vi "main.vi"() -> ()   [LabVIEW 2023]
uses:
  #typedef_state.ctl
  #typedef_caffeetype.ctl
  #typedef_data.ctl
  #typedef_action.ctl
  <vilib>/Utility/file.llb/Write Delimited Spreadsheet (string).vi
panel:
  in  "Caffee Mocha":bool
  in  "Caffee Latte":bool
  in  "Espresso Macchiato":bool
  in  "Espresso":bool
  in  "stop":bool
  out "Whipped Cream":bool
  out "Chocolate Syrup":bool
  out "Milk Foam":bool
  out "Steamed Milk":bool
  out "Espresso":bool
  # "Wybierz kawe:"
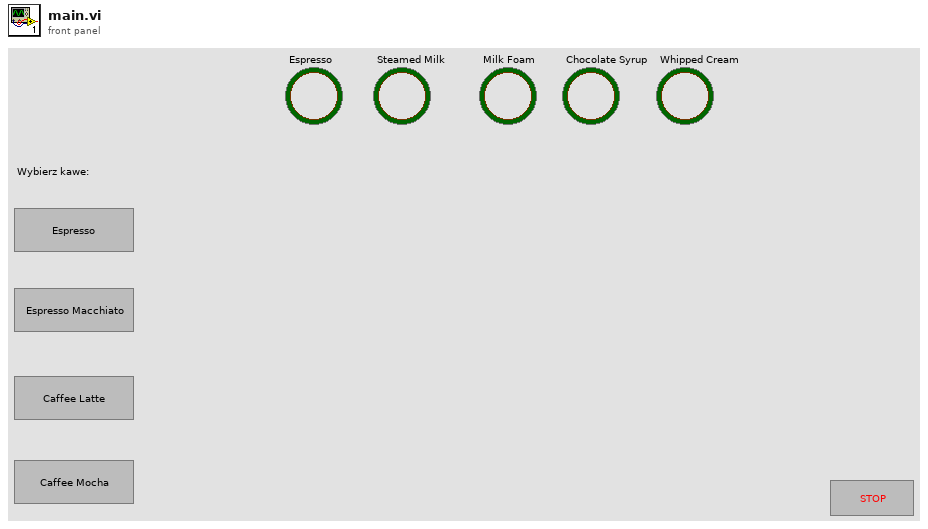
[diagram p1: front panel]
types:
  T1 = typedef "#typedef_caffeetype.ctl" = enum16{"Espresso", "Espresso Macchiato", "Caffee Latte", "Caffee Mocha"}
  T2 = typedef "#typedef_state.ctl" = enum16{"Inicializing", "Idle", "Whipped Cream", "Chocolate Syrup", "Milk Foam", "Steamed Milk", "Espresso", "Stop"}
  T3 = typedef "#typedef_data.ctl" = cluster{"Caffee Type":enum16{"Espresso", "Espresso Macchiato", "Caffee Latte", "Caffee Mocha"}, "Espresso":bool, "Steamed Milk":bool, "Milk Foam":bool, "Chocolate Syrup":bool, "Whipped Cream":bool, "Time reset?":bool}
  T4 = enum16{"Espresso", "Espresso Macchiato", "Caffee Latte", "Caffee Mocha"}
  T5 = typedef "#typedef_action.ctl" = enum16{"Pause", "Reset", "Run"}
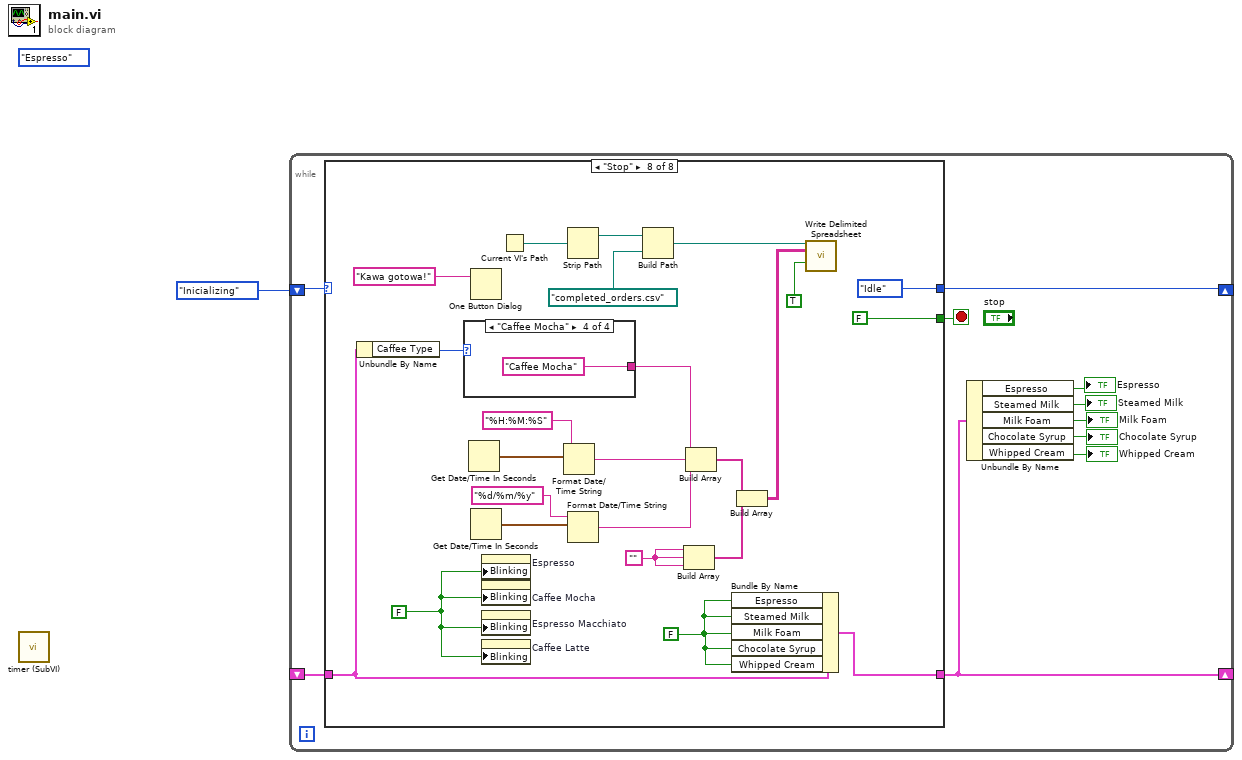
[diagram p0: block diagram]
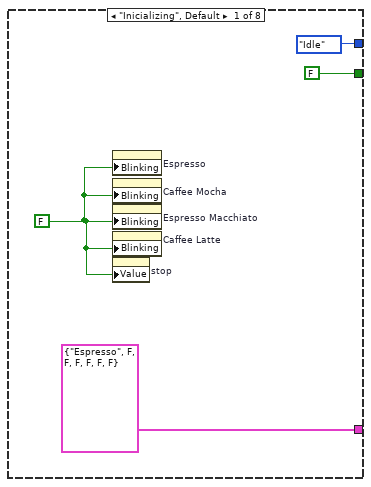
[diagram p2: hidden frame]
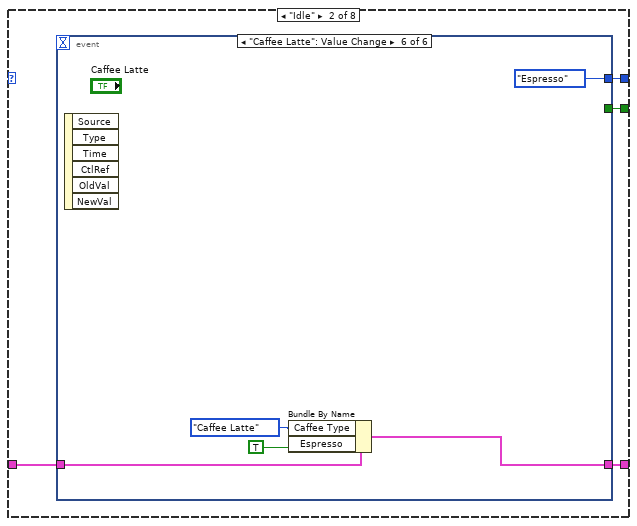
[diagram p3: hidden frame]
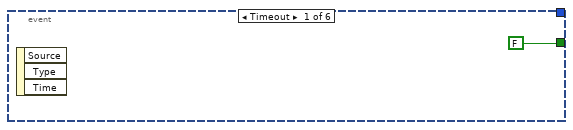
[diagram p4: hidden frame]
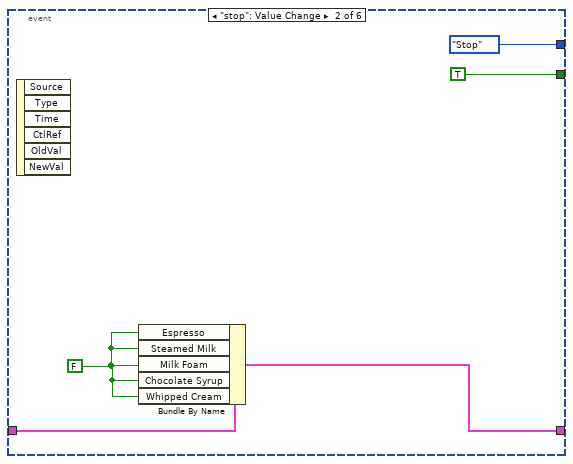
[diagram p5: hidden frame]
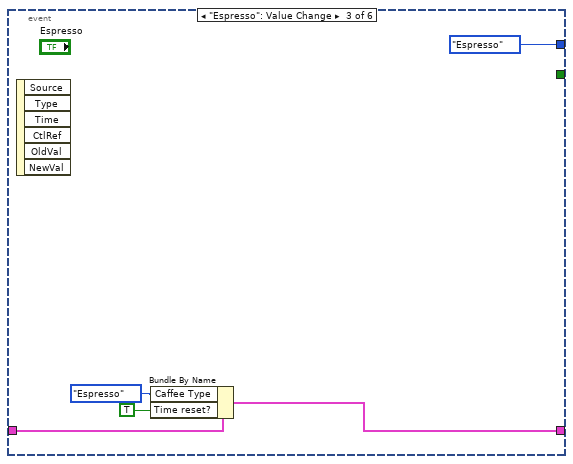
[diagram p6: hidden frame]
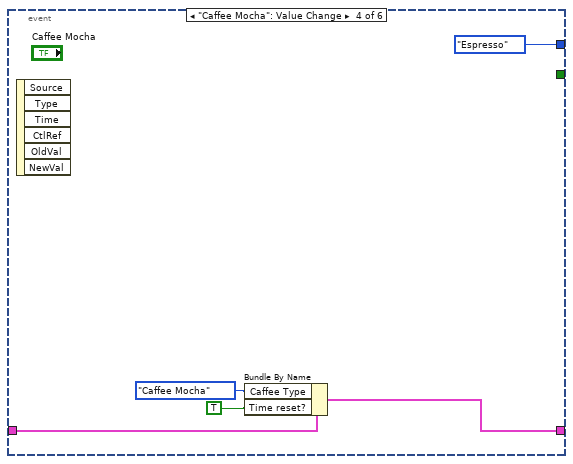
[diagram p7: hidden frame]
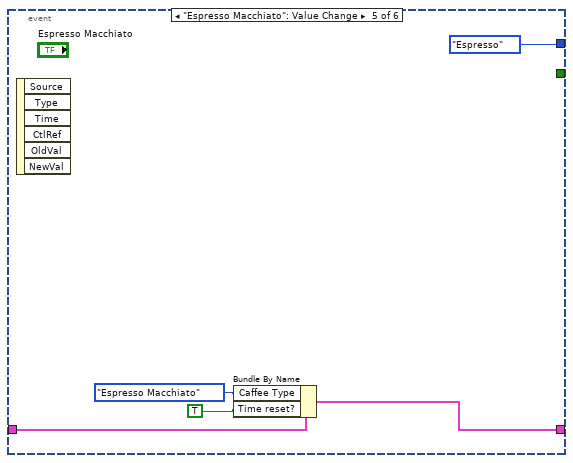
[diagram p8: hidden frame]
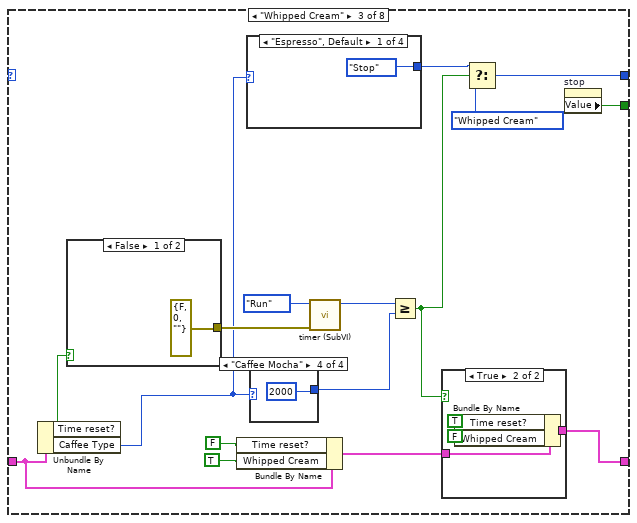
[diagram p9: hidden frame]
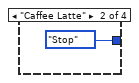
[diagram p11: hidden frame]
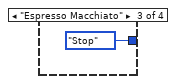
[diagram p12: hidden frame]
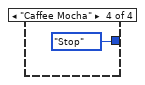
[diagram p13: hidden frame]
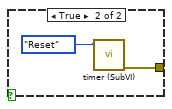
[diagram p14: hidden frame]
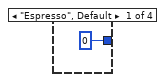
[diagram p15: hidden frame]
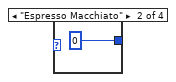
[diagram p16: hidden frame]
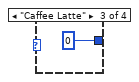
[diagram p17: hidden frame]
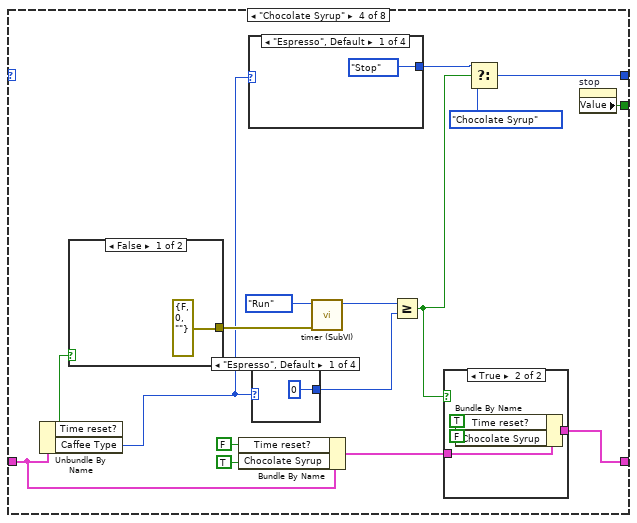
[diagram p18: hidden frame]
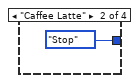
[diagram p20: hidden frame]
diagram:
  (unwired) #typedef_caffeetype."Espresso" ("Caffee Type")
  n1 = call "timer (SubVI).vi"() -> ()  [unwired: 10 in, 2 out]
  n2 = while {
    shift-right: [w10] -> _
    shift-left: #typedef_state."Inicializing" ("State") -> [w11]
    shift-right: [w7] -> _
    shift-left: _ -> [w8]
    stop <- w9 stop-if-true
    n3 = case shown="\"Stop\"" w11 {
      tunnel: [T3 {"Caffee Type"=enum."Espresso", "Espresso"=FALSE, "Steamed Milk"=FALSE, "Milk Foam"=FALSE, "Chocolate Syrup"=FALSE, "Whipped Cream"=FALSE, "Time reset?"=FALSE} ("Data") w16 w49 w80 w114 w144 w177 w230] -> w7
      tunnel: [#typedef_state."Idle" ("State") w18 w51 w82 w115 w146 w183 #typedef_state."Idle" ("State")] -> w10
      tunnel: [FALSE w19 w48 w79 w112 w143 w176 FALSE] -> w9
      tunnel: w8 -> [_ w17 w50 w81 w113 w145 w189 w220]
      frame "Inicializing", Default {
        w12 = FALSE ("stop")
        n4 = property on="Espresso" class="Bool"("Blinking"=w12) -> ()  [unwired: 2 in, 2 out]
        n5 = property on="Caffee Mocha" class="Bool"("Blinking"=w12) -> ()  [unwired: 2 in, 2 out]
        n6 = property on="Espresso Macchiato" class="Bool"("Blinking"=w12) -> ()  [unwired: 2 in, 2 out]
        n7 = property on="Caffee Latte" class="Bool"("Blinking"=w12) -> ()  [unwired: 2 in, 2 out]
        n8 = property on="stop" class="Bool (strict)"("Value"=w12) -> ()  [unwired: 2 in, 2 out]
      }
      frame "Idle" {
        n9 = event shown="[5] \"Caffee Latte\": Value Change" {
          selector: _ -> [_ _ _ _ _ _]
          dyn-events: _ -> [_ _ _ _ _ _]
          timeout: _ -> [_ _ _ _ _ _]
          tunnel: [FALSE TRUE _ _ _ _] -> w19
          tunnel: [_ #typedef_state."Stop" ("State") #typedef_state."Espresso" ("State") #typedef_state."Espresso" ("State") #typedef_state."Espresso" ("State") #typedef_state."Espresso" ("State")] -> w18
          tunnel: w17 -> [_ w23 w29 w33 w39 w44]
          tunnel: [_ w21 w27 w32 w38 w43] -> w16
          event Timeout {
            n10 = event-data() -> ()  [unwired: 1 in, 3 out]
          }
          event "stop": Value Change {
            w22 = FALSE ("Espresso")
            n11 = event-data() -> ()  [unwired: 1 in, 6 out]
            n12 = Bundle By Name(cluster=w23, "Espresso"=w22, "Steamed Milk"=w22, "Milk Foam"=w22, "Chocolate Syrup"=w22, "Whipped Cream"=w22) -> (w21:T3)
          }
          event "Espresso": Value Change {
            n13 = event-data() -> ()  [unwired: 1 in, 6 out]
            n14 = Bundle By Name(cluster=w29, "Caffee Type"=T4."Espresso", "Time reset?"=TRUE) -> (w27:T3)
          }
          event "Caffee Mocha": Value Change {
            n15 = event-data() -> ()  [unwired: 1 in, 6 out]
            n16 = Bundle By Name(cluster=w33, "Caffee Type"=T4."Caffee Mocha", "Time reset?"=TRUE) -> (w32:T3)
          }
          event "Espresso Macchiato": Value Change {
            n17 = event-data() -> ()  [unwired: 1 in, 6 out]
            n18 = Bundle By Name(cluster=w39, "Caffee Type"=T4."Espresso Macchiato", "Time reset?"=TRUE) -> (w38:T3)
          }
          event "Caffee Latte": Value Change {
            n19 = event-data() -> ()  [unwired: 1 in, 6 out]
            n20 = Bundle By Name(cluster=w44, "Caffee Type"=T4."Caffee Latte", "Espresso"=TRUE) -> (w43:T3)
          }
        }
      }
      frame "Whipped Cream" {
        n21 = Unbundle By Name(w50) -> ("Time reset?"=w59:bool, "Caffee Type"=w56:T4)
        n22 = case shown="False" w59 {
          tunnel: [errorcluster {"status"=FALSE, "code"=0, "source"=""} ("error out") w73] -> w61
          frame False {
          }
          frame True {
            n23 = call "timer (SubVI).vi"("Action"=#typedef_action."Reset") -> ("error out"=w73:errorcluster)  [unwired: 9 in, 1 out]
          }
        }
        n24 = Bundle By Name(cluster=w50, "Time reset?"=FALSE, "Whipped Cream"=TRUE) -> (w52:T3)
        n25 = case shown="\"Espresso\", Default" w56 {
          tunnel: [#typedef_state."Stop" ("State") #typedef_state."Stop" ("State") #typedef_state."Stop" ("State") #typedef_state."Stop" ("State")] -> w55
          frame "Espresso", Default {
          }
          frame "Caffee Latte" {
          }
          frame "Espresso Macchiato" {
          }
          frame "Caffee Mocha" {
          }
        }
        n26 = case shown="\"Caffee Mocha\"" w56 {
          tunnel: [0 0 0 2000] -> w58
          frame "Espresso", Default {
          }
          frame "Espresso Macchiato" {
          }
          frame "Caffee Latte" {
          }
          frame "Caffee Mocha" {
          }
        }
        n27 = call "timer (SubVI).vi"("error in (no error)"=w61, "Action"=#typedef_action."Run") -> ("Numeric"=w60:u32)  [unwired: 8 in, 1 out]
        n28 = Greater Or Equal?(x=w60, y=w58) -> (x >= y?=w53:bool)
        n29 = case shown="True" w53 {
          tunnel: w52 -> [w62 w66]
          tunnel: [w62 w63] -> w49
          frame False {
          }
          frame True {
            n30 = Bundle By Name(cluster=w66, "Time reset?"=TRUE, "Whipped Cream"=FALSE ("Espresso")) -> (w63:T3)
          }
        }
        n31 = Select(t=w55, s=w53, f=#typedef_state."Whipped Cream" ("State")) -> (s? t:f=w51:T2)
        n32 = property on="stop" class="Bool (strict)"() -> ("Value"=w48:bool)  [unwired: 2 in, 2 out]
      }
      frame "Chocolate Syrup" {
        n33 = Unbundle By Name(w81) -> ("Time reset?"=w91:bool, "Caffee Type"=w87:T4)
        n34 = case shown="False" w91 {
          tunnel: [errorcluster {"status"=FALSE, "code"=0, "source"=""} ("error out") w105] -> w93
          frame False {
          }
          frame True {
            n35 = call "timer (SubVI).vi"("Action"=#typedef_action."Reset") -> ("error out"=w105:errorcluster)  [unwired: 9 in, 1 out]
          }
        }
        n36 = Bundle By Name(cluster=w81, "Time reset?"=FALSE, "Chocolate Syrup"=TRUE) -> (w83:T3)
        n37 = case shown="\"Espresso\", Default" w87 {
          tunnel: [#typedef_state."Stop" ("State") #typedef_state."Stop" ("State") #typedef_state."Stop" ("State") #typedef_state."Steamed Milk" ("State")] -> w86
          frame "Espresso", Default {
          }
          frame "Caffee Latte" {
          }
          frame "Espresso Macchiato" {
          }
          frame "Caffee Mocha" {
          }
        }
        n38 = case shown="\"Espresso\", Default" w87 {
          tunnel: [0 0 0 2000] -> w89
          frame "Espresso", Default {
          }
          frame "Espresso Macchiato" {
          }
          frame "Caffee Latte" {
          }
          frame "Caffee Mocha" {
          }
        }
        n39 = call "timer (SubVI).vi"("error in (no error)"=w93, "Action"=#typedef_action."Run") -> ("Numeric"=w92:u32)  [unwired: 8 in, 1 out]
        n40 = Greater Or Equal?(x=w92, y=w89) -> (x >= y?=w84:bool)
        n41 = case shown="True" w84 {
          tunnel: w83 -> [w94 w98]
          tunnel: [w94 w95] -> w80
          frame False {
          }
          frame True {
            n42 = Bundle By Name(cluster=w98, "Time reset?"=TRUE, "Chocolate Syrup"=FALSE ("Espresso")) -> (w95:T3)
          }
        }
        n43 = Select(t=w86, s=w84, f=#typedef_state."Chocolate Syrup" ("State")) -> (s? t:f=w82:T2)
        n44 = property on="stop" class="Bool (strict)"() -> ("Value"=w79:bool)  [unwired: 2 in, 2 out]
      }
      frame "Milk Foam" {
        n45 = Unbundle By Name(w113) -> ("Time reset?"=w123:bool, "Caffee Type"=w120:T4)
        n46 = case shown="True" w123 {
          tunnel: [errorcluster {"status"=FALSE, "code"=0, "source"=""} ("error out") w137] -> w125
          frame False {
          }
          frame True {
            n47 = call "timer (SubVI).vi"("Action"=#typedef_action."Reset") -> ("error out"=w137:errorcluster)  [unwired: 9 in, 1 out]
          }
        }
        n48 = case shown="\"Espresso Macchiato\"" w120 {
          tunnel: [#typedef_state."Stop" ("State") #typedef_state."Stop" ("State") #typedef_state."Stop" ("State") #typedef_state."Stop" ("State")] -> w119
          frame "Espresso", Default {
          }
          frame "Caffee Latte" {
          }
          frame "Espresso Macchiato" {
          }
          frame "Caffee Mocha" {
          }
        }
        n49 = case shown="\"Caffee Latte\"" w120 {
          tunnel: [0 2000 2000 0] -> w122
          frame "Espresso", Default {
          }
          frame "Espresso Macchiato" {
          }
          frame "Caffee Latte" {
          }
          frame "Caffee Mocha" {
          }
        }
        n50 = Bundle By Name(cluster=w113, "Time reset?"=FALSE, "Milk Foam"=TRUE) -> (w116:T3)
        n51 = call "timer (SubVI).vi"("error in (no error)"=w125, "Action"=#typedef_action."Run") -> ("Numeric"=w124:u32)  [unwired: 8 in, 1 out]
        n52 = Greater Or Equal?(x=w124, y=w122) -> (x >= y?=w117:bool)
        n53 = case shown="True" w117 {
          tunnel: w116 -> [w126 w130]
          tunnel: [w126 w127] -> w114
          frame False {
          }
          frame True {
            n54 = Bundle By Name(cluster=w130, "Time reset?"=TRUE, "Milk Foam"=FALSE ("Espresso")) -> (w127:T3)
          }
        }
        n55 = Select(t=w119, s=w117, f=#typedef_state."Milk Foam" ("State")) -> (s? t:f=w115:T2)
        n56 = property on="stop" class="Bool (strict)"() -> ("Value"=w112:bool)  [unwired: 2 in, 2 out]
      }
      frame "Steamed Milk" {
        n57 = Unbundle By Name(w145) -> ("Time reset?"=w155:bool, "Caffee Type"=w151:T4)
        n58 = case shown="True" w155 {
          tunnel: [errorcluster {"status"=FALSE, "code"=0, "source"=""} ("error out") w169] -> w157
          frame False {
          }
          frame True {
            n59 = call "timer (SubVI).vi"("Action"=#typedef_action."Reset") -> ("error out"=w169:errorcluster)  [unwired: 9 in, 1 out]
          }
        }
        n60 = Bundle By Name(cluster=w145, "Time reset?"=FALSE, "Steamed Milk"=TRUE) -> (w147:T3)
        n61 = case shown="\"Caffee Latte\"" w151 {
          tunnel: [0 0 8000 2000] -> w153
          frame "Espresso", Default {
          }
          frame "Espresso Macchiato" {
          }
          frame "Caffee Latte" {
          }
          frame "Caffee Mocha" {
          }
        }
        n62 = case shown="\"Caffee Latte\"" w151 {
          tunnel: [#typedef_state."Stop" ("State") #typedef_state."Milk Foam" ("State") #typedef_state."Stop" ("State") #typedef_state."Whipped Cream" ("State")] -> w150
          frame "Espresso", Default {
          }
          frame "Caffee Latte" {
          }
          frame "Espresso Macchiato" {
          }
          frame "Caffee Mocha" {
          }
        }
        n63 = call "timer (SubVI).vi"("error in (no error)"=w157, "Action"=#typedef_action."Run") -> ("Numeric"=w156:u32)  [unwired: 8 in, 1 out]
        n64 = Greater Or Equal?(x=w156, y=w153) -> (x >= y?=w148:bool)
        n65 = case shown="True" w148 {
          tunnel: w147 -> [w158 w162]
          tunnel: [w158 w159] -> w144
          frame False {
          }
          frame True {
            n66 = Bundle By Name(cluster=w162, "Time reset?"=TRUE, "Steamed Milk"=FALSE ("Espresso")) -> (w159:T3)
          }
        }
        n67 = Select(t=w150, s=w148, f=#typedef_state."Steamed Milk" ("State")) -> (s? t:f=w146:T2)
        n68 = property on="stop" class="Bool (strict)"() -> ("Value"=w143:bool)  [unwired: 2 in, 2 out]
      }
      frame "Espresso" {
        n69 = Unbundle By Name(w189) -> ("Time reset?"=w186:bool, "Caffee Type"=w175:T4)
        n70 = case shown="True" w186 {
          tunnel: [errorcluster {"status"=FALSE, "code"=0, "source"=""} ("error out") w205] -> w188
          frame False {
          }
          frame True {
            n71 = call "timer (SubVI).vi"("Action"=#typedef_action."Reset") -> ("error out"=w205:errorcluster)  [unwired: 9 in, 1 out]
          }
        }
        n72 = case shown="\"Espresso\", Default" w175 {
          tunnel: [#typedef_state."Stop" ("State") #typedef_state."Steamed Milk" ("State") #typedef_state."Milk Foam" ("State") #typedef_state."Chocolate Syrup" ("State")] -> w181
          frame "Espresso", Default {
          }
          frame "Caffee Latte" {
          }
          frame "Espresso Macchiato" {
          }
          frame "Caffee Mocha" {
          }
        }
        n73 = case shown="\"Espresso\", Default" w175 {
          tunnel: [6000 6000 5000 5000] -> w184
          frame "Espresso", Default {
          }
          frame "Espresso Macchiato" {
          }
          frame "Caffee Latte" {
          }
          frame "Caffee Mocha" {
          }
        }
        n74 = Bundle By Name(cluster=w189, "Time reset?"=FALSE, "Espresso"=TRUE) -> (w178:T3)
        n75 = case shown="\"Caffee Mocha\"" w175 {
          frame "Espresso", Default {
            n76 = property on="Espresso" class="Bool"("Blinking"=TRUE) -> ()  [unwired: 2 in, 2 out]
          }
          frame "Espresso Macchiato" {
            n77 = property on="Espresso Macchiato" class="Bool"("Blinking"=TRUE) -> ()  [unwired: 2 in, 2 out]
          }
          frame "Caffee Latte" {
            n78 = property on="Caffee Latte" class="Bool"("Blinking"=TRUE) -> ()  [unwired: 2 in, 2 out]
          }
          frame "Caffee Mocha" {
            n79 = property on="Caffee Mocha" class="Bool"("Blinking"=TRUE) -> ()  [unwired: 2 in, 2 out]
          }
        }
        n80 = call "timer (SubVI).vi"("error in (no error)"=w188, "Action"=#typedef_action."Run") -> ("Numeric"=w187:u32)  [unwired: 8 in, 1 out]
        n81 = Greater Or Equal?(x=w187, y=w184) -> (x >= y?=w179:bool)
        n82 = case shown="True" w179 {
          tunnel: w178 -> [w194 w198]
          tunnel: [w194 w195] -> w177
          frame False {
          }
          frame True {
            n83 = Bundle By Name(cluster=w198, "Time reset?"=TRUE, "Espresso"=FALSE) -> (w195:T3)
          }
        }
        n84 = Select(t=w181, s=w179, f=#typedef_state."Espresso" ("State")) -> (s? t:f=w183:T2)
        n85 = property on="stop" class="Bool (strict)"() -> ("Value"=w176:bool)  [unwired: 2 in, 2 out]
      }
      frame "Stop" {
        w210 = FALSE ("Blinking")
        w215 = ""
        w231 = FALSE ("Espresso")
        n86 = Unbundle By Name(w220) -> ("Caffee Type"=w219:T4)
        n87 = case shown="\"Caffee Mocha\"" w219 {
          tunnel: ["Espresso" " Espresso Macchiato\"" "Caffee Latte" "Caffee Mocha"] -> w216
          frame "Espresso", Default {
          }
          frame "Espresso Macchiato" {
          }
          frame "Caffee Latte" {
          }
          frame "Caffee Mocha" {
          }
        }
        n88 = Get Date/Time In Seconds() -> (seconds since 1Jan1904=w225:timestamp)
        n89 = One Button Dialog(message="Kawa gotowa!") -> ()  [unwired: 1 in, 1 out]
        n90 = Get Date/Time In Seconds() -> (seconds since 1Jan1904=w224:timestamp)
        n91 = property on="Espresso" class="Bool"("Blinking"=w210) -> ()  [unwired: 2 in, 2 out]
        n92 = property on="Caffee Mocha" class="Bool"("Blinking"=w210) -> ()  [unwired: 2 in, 2 out]
        n93 = property on="Espresso Macchiato" class="Bool"("Blinking"=w210) -> ()  [unwired: 2 in, 2 out]
        n94 = property on="Caffee Latte" class="Bool"("Blinking"=w210) -> ()  [unwired: 2 in, 2 out]
        n95 = Current VI's Path() -> (path=w228:path)
        n96 = Format Date/Time String(time format string (%c)="%H:%M:%S", seconds (now)=w225) -> (date/time string=w217:string)  [unwired: 1 in]
        n97 = Strip Path(path=w228) -> (stripped path=w227:path)  [unwired: 1 out]
        n98 = Format Date/Time String(time format string (%c)="%d/%m/%y", seconds (now)=w224) -> (date/time string=w218:string)  [unwired: 1 in]
        n99 = Build Path(base path=w227, name or relative path=path "completed_orders.csv") -> (appended path=w226:path)
        n100 = Build Array(w215, w215, w215) -> (w213:string[])
        n101 = Build Array(w216, w217, w218) -> (w214:string[])
        n102 = Bundle By Name(cluster=w220, "Espresso"=w231, "Steamed Milk"=w231, "Milk Foam"=w231, "Chocolate Syrup"=w231, "Whipped Cream"=w231) -> (w230:T3)
        n103 = Build Array(w214, w213) -> (w212:string[][])
        n104 = call-poly <vilib>:"Write Delimited Spreadsheet.vi"("file path (dialog if empty)"=w226, "2D data"=w212, "append to file? (new file:F)"=TRUE) -> ()  [unwired: 11 in, 2 out]
      }
    }
    n105 = Unbundle By Name(w7) -> ("Espresso"=→"Espresso":bool, "Steamed Milk"=→"Steamed Milk":bool, "Milk Foam"=→"Milk Foam":bool, "Chocolate Syrup"=→"Chocolate Syrup":bool, "Whipped Cream"=→"Whipped Cream":bool)
  }
